vi "heating_visu_colors.vi"(10 "Z_State":T1=enum."on", 11 "Z_Source":T2=enum."local disabled") -> (0 "slide visible":bool, 1 "on visible":bool, 2 "auto visible":bool, 3 "N ring":u16)   [LabVIEW 2019, in "Heating.lvlib"]
uses:
  Heating.lvlib
  ctl/Y_source.ctl
  ctl/Z_State.ctl
  Counter/Counter.lvlib
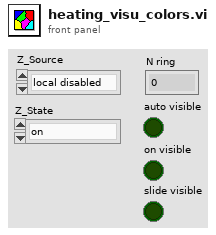
[diagram p1: front panel]
types:
  T1 = typedef "Heating.lvlib/Z_State.ctl" = enum8{"initialization", "alarm", "disabled", "not ready", "stop ready", "reserv", "switched off", "reserv2", "switched on", "check", "on min", "decrease out", "on", "increase out", "on max"}
  T2 = typedef "Heating.lvlib/Y_source.ctl" = enum8{"initialize", "local disabled", "local hand", "hand", "auto", "dist"}
  T3 = enum8{"local disabled", "local hand", "hand", "auto", "dist"}
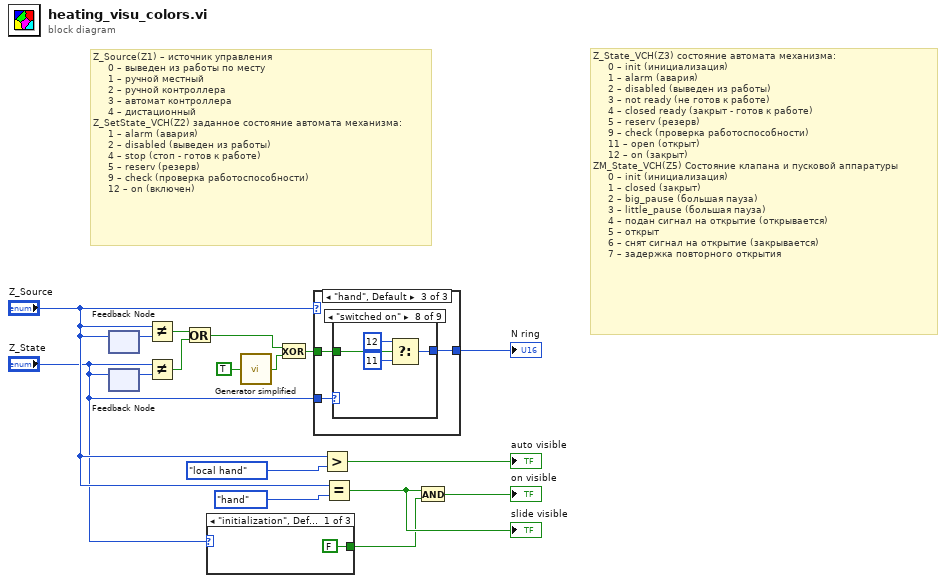
[diagram p0: block diagram]
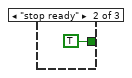
[diagram p2: hidden frame]
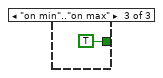
[diagram p3: hidden frame]
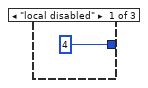
[diagram p4: hidden frame]
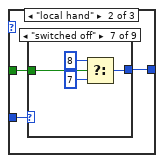
[diagram p5: hidden frame]
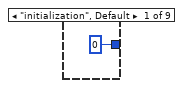
[diagram p6: hidden frame]
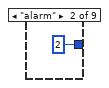
[diagram p7: hidden frame]
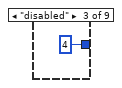
[diagram p8: hidden frame]
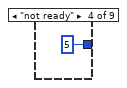
[diagram p9: hidden frame]
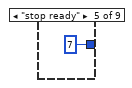
[diagram p10: hidden frame]
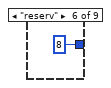
[diagram p11: hidden frame]
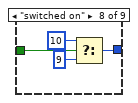
[diagram p12: hidden frame]
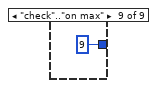
[diagram p13: hidden frame]
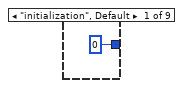
[diagram p14: hidden frame]
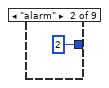
[diagram p15: hidden frame]
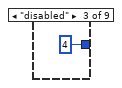
[diagram p16: hidden frame]
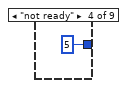
[diagram p17: hidden frame]
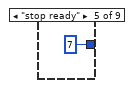
[diagram p18: hidden frame]
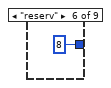
[diagram p19: hidden frame]
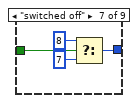
[diagram p20: hidden frame]
diagram:
  # "Z_State_VCH(Z3) состояние автомата механизма:\n     0 – init (инициализация)\n     1 – alarm (авария)\n     2 – disabled (выведен из работы)\n     3 – not ready (не готов к работе)\n     4 – closed ready (закрыт - готов к работе)\n     5 – reserv (резерв)\n     9 – check (проверка работоспособности)\n     11 – open (открыт)\n     12 – on (закрыт)\nZM_State_VCH(Z5) Состояние клапана и пусковой аппаратуры\n     0 – init (инициализация)\n     1 – сlosed (закрыт)\n     2 – big_pause (большая пауза)\n     3 – little_pause (большая пауза)\n     4 – подан сигнал на открытие (открывается)\n     5 – открыт\n     6 – снят сигнал на открытие (закрывается)\n     7 – задержка повторного открытия"
  # "Z_Source(Z1) – источник управления\n     0 – выведен из работы по месту\n     1 – ручной местный\n     2 – ручной контроллера\n     3 – автомат контроллера\n     4 – дистационный\nZ_SetState_VCH(Z2) заданное состояние автомата механизма:\n     1 – alarm (авария)\n     2 – disabled (выведен из работы)\n     4 – stop (стоп - готов к работе)\n     5 – reserv (резерв)\n     9 – check (проверка работоспособности)\n     12 – on (включен)"
  n1 = feedback #1() -> (w17:T2)  [unwired: 1 in]
  n2 = feedback-in #1("Z_Source") -> ()
  n3 = feedback #2() -> (w16:T1)  [unwired: 1 in]
  n4 = feedback-in #2("Z_State") -> ()
  n5 = Not Equal?(x="Z_Source", y=w17) -> (x != y?=w15:bool)
  n6 = Not Equal?(x="Z_State", y=w16) -> (x != y?=w14:bool)
  n7 = Or(x=w15, y=w14) -> (x .or. y?=w1:bool)
  n8 = case shown="\"initialization\", Default" "Z_State" {
    tunnel: [FALSE TRUE TRUE] -> w6
    frame "initialization", Default {
    }
    frame "stop ready" {
    }
    frame "on min".."on max" {
    }
  }
  n9 = call "Generator simplified.vi"("ON (F)"=TRUE) -> ("Q"=w3:bool)
  n10 = Exclusive Or(1:w3, 2:w1) -> (0:w2:bool)
  n11 = case shown="\"hand\", Default" "Z_Source" {
    tunnel: w2 -> [_ w24 w41]
    tunnel: "Z_State" -> [_ w23 w42]
    tunnel: [u16 4 ("Z5 ind") w22 w40] -> w13
    frame "local disabled" {
    }
    frame "local hand" {
      n12 = case shown="\"switched off\"" w23 {
        tunnel: [u16 0 ("Z5 ind") u16 2 ("Z5 ind") u16 4 ("Z5 ind") u16 5 ("Z5 ind") u16 7 ("Z5 ind") u16 8 ("Z5 ind") w32 w36 u16 9 ("Z5 ind")] -> w22
        tunnel: w24 -> [_ _ _ _ _ _ w31 w35 _]
        frame "initialization", Default {
        }
        frame "alarm" {
        }
        frame "disabled" {
        }
        frame "not ready" {
        }
        frame "stop ready" {
        }
        frame "reserv" {
        }
        frame "switched off" {
          n13 = Select(t=u16 8 ("Z5 ind"), s=w31, f=u16 7) -> (s? t:f=w32:u16)
        }
        frame "switched on" {
          n14 = Select(t=u16 10 ("Z5 ind"), s=w35, f=u16 9) -> (s? t:f=w36:u16)
        }
        frame "check".."on max" {
        }
      }
    }
    frame "hand", Default {
      n15 = case shown="\"switched on\"" w42 {
        tunnel: [u16 0 ("Z5 ind") u16 2 ("Z5 ind") u16 4 ("Z5 ind") u16 5 ("Z5 ind") u16 7 ("Z5 ind") u16 8 ("Z5 ind") w50 w54 u16 11 ("Z5 ind")] -> w40
        tunnel: w41 -> [_ _ _ _ _ _ w49 w53 _]
        frame "initialization", Default {
        }
        frame "alarm" {
        }
        frame "disabled" {
        }
        frame "not ready" {
        }
        frame "stop ready" {
        }
        frame "reserv" {
        }
        frame "switched off" {
          n16 = Select(t=u16 8 ("Z5 ind"), s=w49, f=u16 7) -> (s? t:f=w50:u16)
        }
        frame "switched on" {
          n17 = Select(t=u16 12 ("Z5 ind"), s=w53, f=u16 11) -> (s? t:f=w54:u16)
        }
        frame "check".."on max" {
        }
      }
    }
  }
  "N ring" <- w13
  n18 = Greater?(x="Z_Source", y=T3."local hand" ("Z1(CmdSource) 2")) -> (0:→"auto visible":bool)
  n19 = Equal?(x="Z_Source", y=T3."hand" ("Z1(CmdSource) 2")) -> (x = y?=w10:bool)
  "slide visible" <- w10
  n20 = And(x=w10, y=w6) -> (x .and. y?=→"on visible":bool)
